vi "uc480_SubVI_Example_CameraInit.vi"(8 "Error In":errorcluster, 9 "Camera ID":i32, 10 "Init Camera Flag":bool, 11 ".NET (Reference)":refnum<k24>) -> (0 "Error Out":errorcluster, 3 ".NET (Reference)":refnum<k24>)   [LabVIEW 2016]
uses:
  D:/Fabrizio/Labview Projects/IR OPO Controller/Branches/Schwarzschild version/uc480DotNet.dll
  uc480DotNet.dll
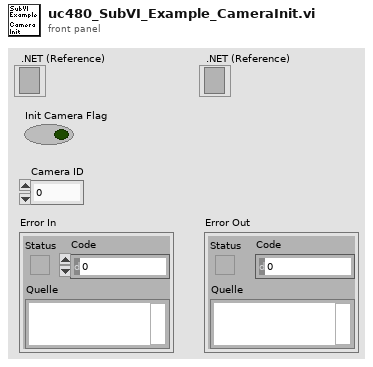
[diagram p1: front panel]
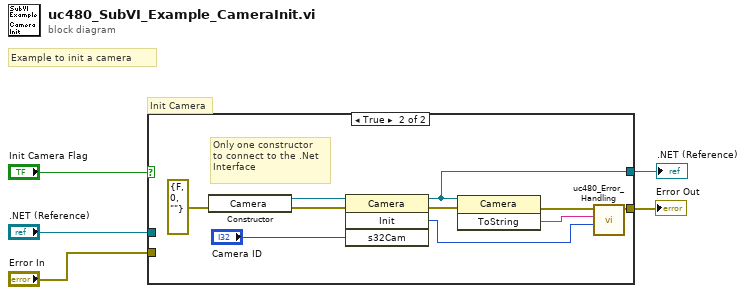
[diagram p0: block diagram]
diagram:
  # "Example to init a camera"
  # "Init Camera"
  n1 = case shown="True" "Init Camera Flag" {
    tunnel: [w6 w10] -> w2
    tunnel: [w7 w8] -> w1
    tunnel: ".NET (Reference)" -> [w7 _]
    tunnel: "Error In" -> [w6 _]
    frame False {
    }
    frame True {
      # "Only one constructor\nto connect to the .Net\nInterface"
      n2 = constructor class="Camera"(error in=errorcluster {"status"=FALSE, "code"=0, "source"=""} ("error in (no error)")) -> (reference out=w15:refnum<k24>, error out=w17:errorcluster)  [unwired: 2 in, 1 out]
      n3 = invoke class="Camera" method="Init"(reference=w15, error in=w17, "s32Cam"="Camera ID") -> (reference out=w8:refnum<k24>, error out=w13:errorcluster, "Init"=w12:i32)  [unwired: 1 in, 1 out]
      n4 = invoke class="Camera" method="ToString"(reference=w8, error in=w13) -> (error out=w14:errorcluster, "ToString"=w11:string)  [unwired: 1 in, 1 out]
      n5 = call "uc480_Error_Handling.vi"("Error Code"=w12, "Error String"=w11, "Error In"=w14) -> ("Error Out"=w10:errorcluster)  [unwired: 8 in]
    }
  }
  ".NET (Reference)" <- w1
  "Error Out" <- w2
